vi "N5765A_Get Power Supplies.vi"(11 "PS_Settings":T1[](array[typedef])) -> (3 "Power Supplies":string[](array[string]))   [LabVIEW 2015]
uses:
  N5765A_PS_Settings.ctl
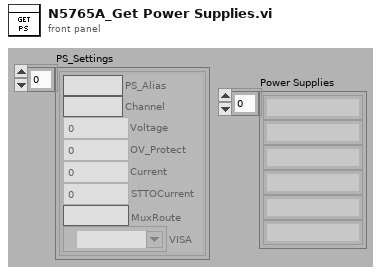
[diagram p1: front panel]
types:
  T1 = typedef "N5765A_PS_Settings.ctl" = cluster{"PS_Alias":string, "Channel":string, "Voltage":dbl, "OV_Protect":dbl, "Current":dbl, "STTOCurrent":dbl, "MuxRoute":string, "VISA":refnum<visa-resource-name>}
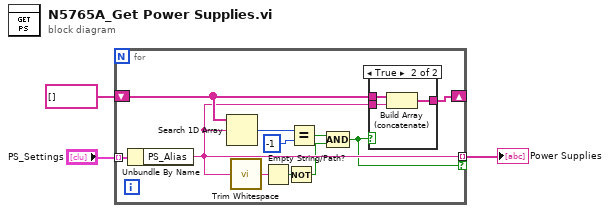
[diagram p0: block diagram]
diagram:
  n1 = for {
    tunnel: "PS_Settings" -> [w14] mode=indexing
    tunnel: [w9] -> w1 mode=indexing if=w5
    shift-right: [w11] -> _
    shift-left: string[] [] ("Array 2") -> [w12]
    n2 = Unbundle By Name(w14) -> ("PS_Alias"=w9:string)
    n3 = Search 1D Array(1D array=w12, element=w9) -> (index of element=w10:i32)  [unwired: 1 in]
    n4 = call <vilib>:"Trim Whitespace.vi"("string"=w9) -> ("trimmed string"=w8:string)  [unwired: 1 in]
    n5 = Empty String/Path?(string/path=w8) -> (empty?=w7:bool)
    n6 = Not(x=w7) -> (.not. x?=w4:bool)
    n7 = Equal?(x=w10, y=-1) -> (x = y?=w6:bool)
    n8 = Compound Arithmetic op=AND(w6, w4) -> (w5:bool)
    n9 = case shown="True" w5 {
      tunnel: w12 -> [w15 w18]
      tunnel: w9 -> [_ w17]
      tunnel: [w15 w16] -> w11
      frame False {
      }
      frame True {
        n10 = Build Array (concatenate)(w18, w17) -> (w16:string[])
      }
    }
  }
  "Power Supplies" <- w1
